vi "Cast FXP to I32.vi"(4 "Array in":fxp<+/-,22,22>[](array[numeric])) -> (1 "Array out":i32[](array[numeric]))   [LabVIEW 2015]
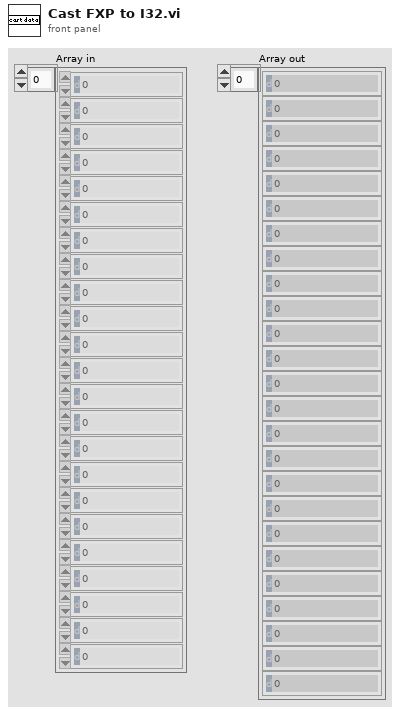
[diagram p1: front panel]
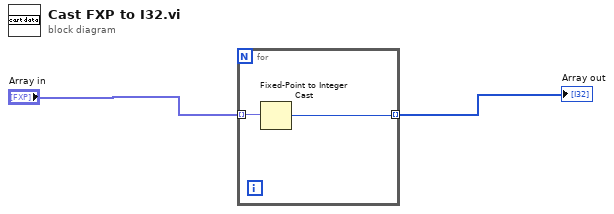
[diagram p0: block diagram]
diagram:
  n1 = for {
    tunnel: "Array in" -> [w4] mode=indexing
    tunnel: [w3] -> w1 mode=indexing
    n2 = Fixed-Point to Integer Cast(1:w4) -> (0:w3:i32)
  }
  "Array out" <- w1
